vi "Sine_wave R2.vi"() -> ()   [LabVIEW 2018]
uses:
  <vilib>/measure/NI_MABase.lvlib
panel:
  out "Y":dbl[](array[numeric])
  out "dt":dbl
  out "t0":timestamp
  in  "Stop Button":bool
  in  "sampling info":cluster{"Fs":dbl, "#s":dbl}={"Fs"=1000.0, "#s"=1000.0} {"Fs" format="%.2p"}
  out "Waveform Graph":waveform(dbl)(graph)
  in  "amplitude\n[V]":dbl
  in  "Frequency \n[1/s]":dbl
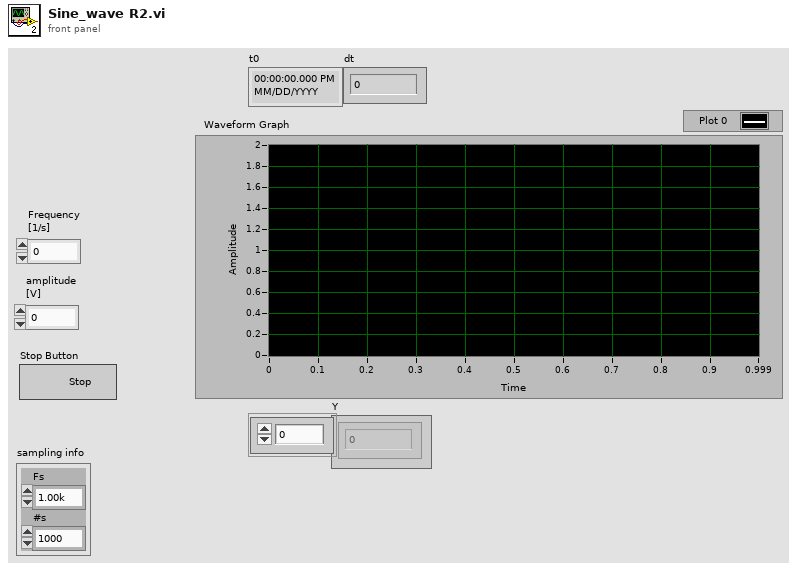
[diagram p1: front panel]
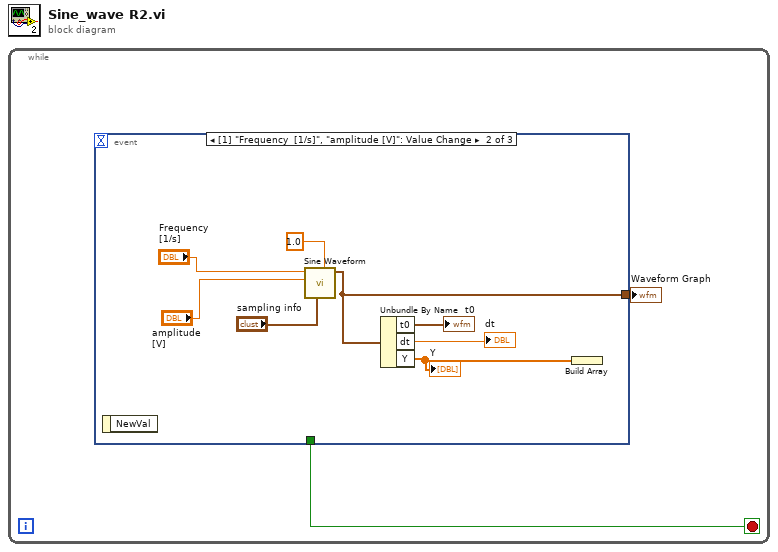
[diagram p0: block diagram]
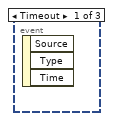
[diagram p2: hidden frame]
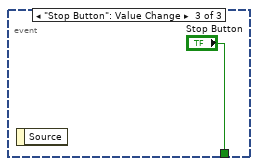
[diagram p3: hidden frame]
diagram:
  n1 = while {
    stop <- w2 stop-if-true
    n2 = event shown="[1] \"Frequency  [1/s]\", \"amplitude [V]\": Value Change" {
      selector: _ -> [_ _ _]
      dyn-events: _ -> [_ _ _]
      timeout: _ -> [_ _ _]
      tunnel: [_ w7 _] -> w1
      tunnel: [_ _ "Stop Button"] -> w2
      event Timeout {
        n3 = event-data() -> ()  [unwired: 1 in, 3 out]
      }
      event "Frequency \n[1/s]", "amplitude\n[V]": Value Change {
        n4 = event-data() -> ()  [unwired: 1 in, 1 out]
        n5 = call <vilib>:"Sine Waveform.vi"("offset"=1.0, "sampling info"="sampling info", "amplitude"="amplitude\n[V]", "frequency"="Frequency \n[1/s]") -> ("signal out"=w7:waveform(dbl))  [unwired: 6 in, 1 out]
        n6 = Unbundle By Name(w7) -> ("t0"=→"t0":timestamp, "dt"=→"dt":dbl, "Y"=w4:dbl[])
        "Y" <- w4
        n7 = Build Array(w4) -> ()  [unwired: 1 out]
      }
      event "Stop Button": Value Change {
        n8 = event-data() -> ()  [unwired: 1 in, 1 out]
      }
    }
    "Waveform Graph" <- w1
  }
